vi "RT TDMS buffer and interpolate.vi"(0 "State Info":T4, 7 "TDMS config":T1, 11 "error in":errorcluster, 13 "Operation":T3(ring)) -> (4 "State Info out":T2, 15 "error out":errorcluster)   [LabVIEW 2010, in "TDMS Custom Device.lvlib"]
uses:
  TDMS Custom Device.lvlib
  <vilib>/Analysis/NI_AALPro.lvlib
  <vilib>/gmath/NI_Gmath.lvlib
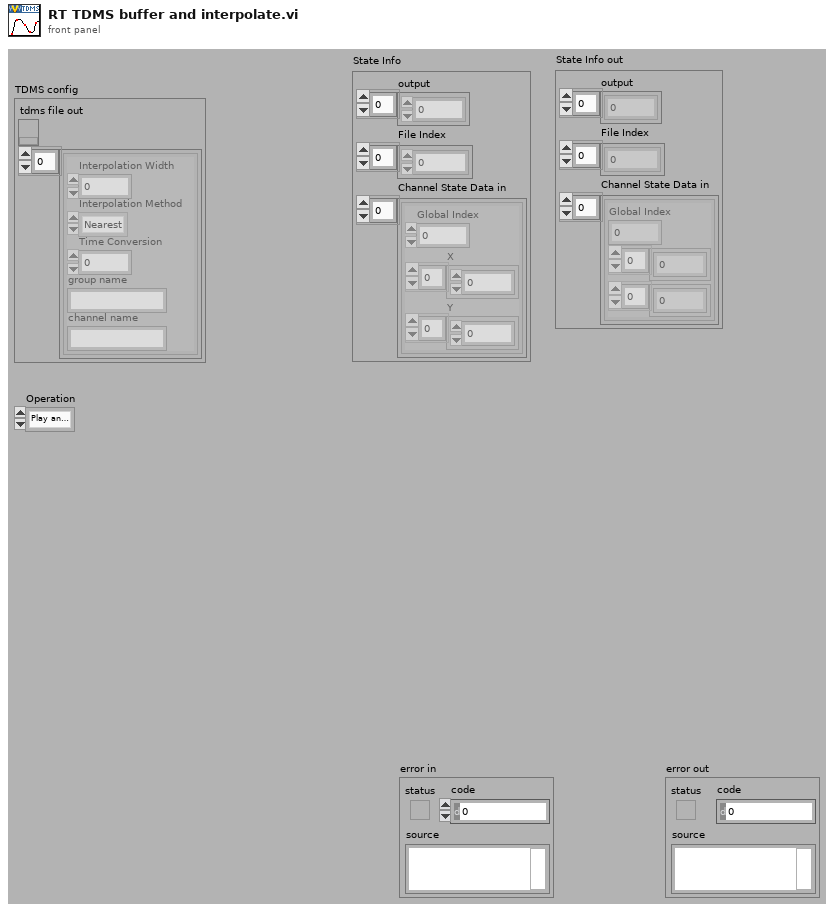
[diagram p1: front panel]
types:
  T1 = cluster{"tdms file out":refnum<k34>, cluster{"Interpolation Width":i32, "Interpolation Method":enum16{"Nearest", "Linear", "Spline", "Cubic Hermite", "Lagrange", "Polynomial"}, "Time Conversion":dbl, "group name":string, "channel name":string}[]}
  T2 = cluster{"output":dbl[], "File Index":i64[], "Channel State Data in":cluster{"Global Index":i64, dbl[], dbl[]}[]}
  T3 = enum16{"Play and Repeat Last", "Stop (and Reset)", "Loop", "Pause"}
  T4 = cluster{"output":dbl[], "File Index":i64[], "Channel State Data in":cluster{"Global Index":i64, "X":dbl[], "Y":dbl[]}[]}
  T5 = cluster{"Global Index":i64, "X":dbl[], "Y":dbl[]}[]
  T6 = cluster{"Interpolation Width":i32, "Interpolation Method":enum16{"Nearest", "Linear", "Spline", "Cubic Hermite", "Lagrange", "Polynomial"}, "Time Conversion":dbl, "group name":string, "channel name":string}[]
  T7 = enum16{"Nearest", "Linear", "Spline", "Cubic Hermite", "Lagrange", "Polynomial"}
  T8 = cluster{"Global Index":i64, "X":dbl[], "Y":dbl[]}
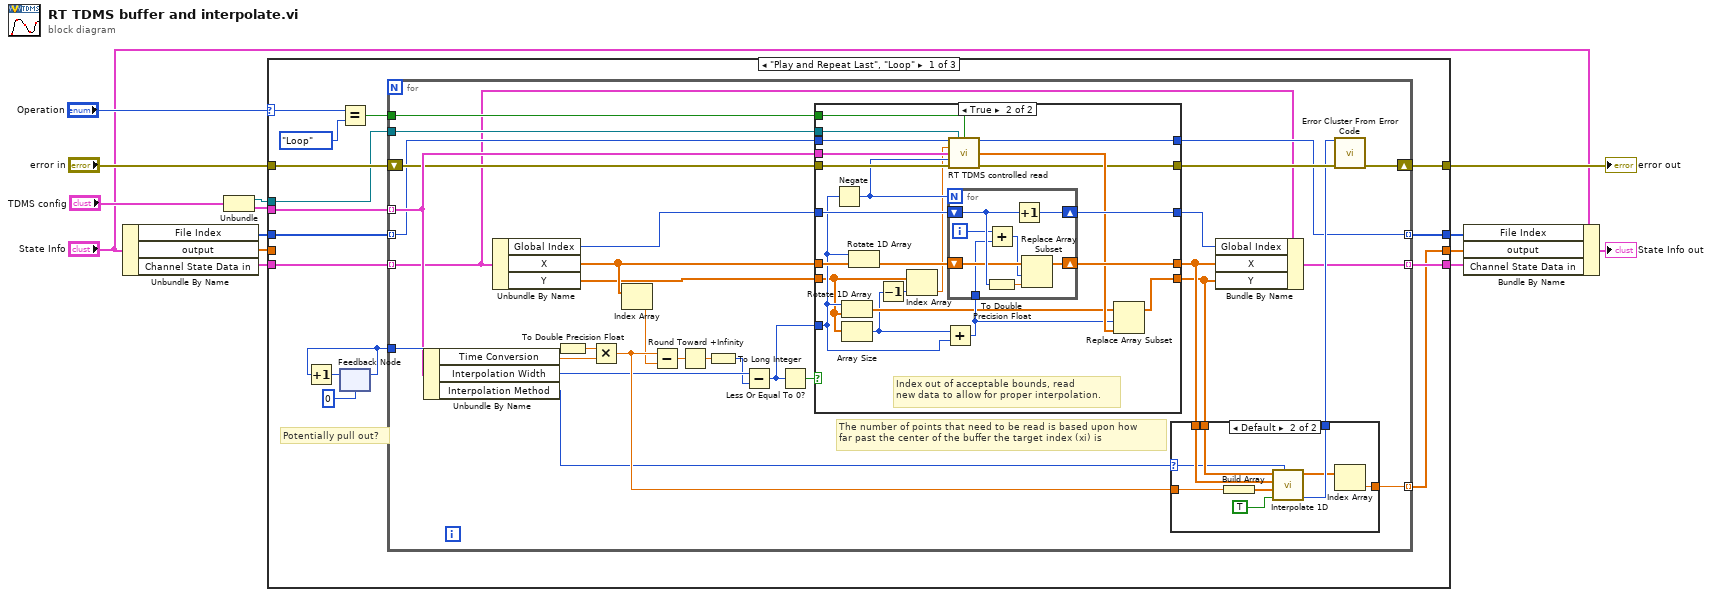
[diagram p0: block diagram]
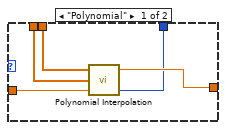
[diagram p2: hidden frame]
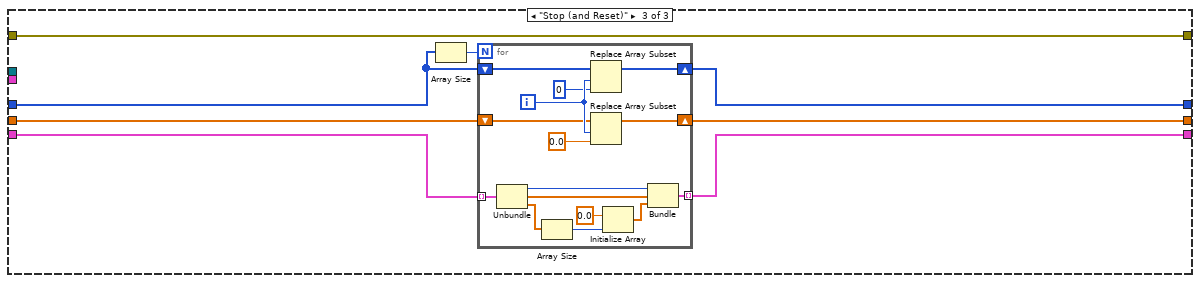
[diagram p5: hidden frame]
diagram:
  n1 = Unbundle By Name("State Info") -> ("File Index"=w8:i64[], "output"=w9:dbl[], "Channel State Data in"=w10:T5)
  n2 = Unbundle("TDMS config") -> ("tdms file out"=w1:refnum<k34>, w2:T6)
  n3 = case shown="\"Play and Repeat Last\", \"Loop\"" "Operation" {
    selector: "Operation" -> [w20 _ _]
    tunnel: "error in" -> [w29 w109 w120]
    tunnel: [w28 w109 w120] -> w13
    tunnel: w9 -> [_ w111 w119]
    tunnel: w2 -> [w27 _ _]
    tunnel: w1 -> [w26 _ _]
    tunnel: w8 -> [w17 w112 w117]
    tunnel: w10 -> [w25 w110 w114]
    tunnel: [w24 w110 w113] -> w7
    tunnel: [w15 w111 w116] -> w3
    tunnel: [w16 w112 w115] -> w4
    frame "Play and Repeat Last", "Loop" {
      # "Potentially pull out?"
      n4 = Equal?(x=w20, y=T3."Loop" ("element")) -> (x = y?=w18:bool)
      n5 = feedback #1(i64 0 ("System Time Index 2")) -> (w21:i64)
      n6 = Increment(x=w21) -> (x+1=w22:i64)
      n7 = feedback-in #1(w22) -> ()
      n8 = for {
        tunnel: w25 -> [w36] mode=indexing
        tunnel: w21 -> [w59]
        tunnel: w27 -> [w56] mode=indexing
        tunnel: [w57] -> w15 mode=indexing
        shift-right: [w53] -> w28
        shift-left: w29 -> [w55]
        tunnel: w26 -> [w51]
        tunnel: w17 -> [w50] mode=indexing
        tunnel: [w35] -> w24 mode=indexing
        tunnel: [w48] -> w16 mode=indexing
        tunnel: w18 -> [w49]
        # "The number of points that need to be read is based upon how\nfar past the center of the buffer the target index (xi) is"
        n9 = Unbundle By Name(w56) -> ("Time Conversion"=w45:dbl, "Interpolation Width"=w31:i32, "Interpolation Method"=w42:T7)
        n10 = Unbundle By Name(w36) -> ("Global Index"=w39:i64, "X"=w38:dbl[], "Y"=w37:dbl[])
        n11 = To Double Precision Float(number=w59) -> (double precision float=w58:dbl)
        n12 = Multiply(x=w58, y=w45) -> (x*y=w47:dbl)
        n13 = Index Array(array=w38) -> (element=w46:dbl)  [unwired: 1 in]
        n14 = Subtract(x=w47, y=w46) -> (x-y=w44:dbl)
        n15 = Round Toward +Infinity(x=w44) -> (ceil(x): smallest int >= x=w43:dbl)
        n16 = To Long Integer(number=w43) -> (32bit integer=w30:i32)
        n17 = Subtract(x=w31, y=w30) -> (x-y=w40:i32)
        n18 = Less Or Equal To 0?(x=w40) -> (x <= 0?=w41:bool)
        n19 = case shown="True" w41 {
          tunnel: w37 -> [w78 w82]
          tunnel: [w74 w100] -> w33
          tunnel: [w78 w99] -> w32
          tunnel: [w75 w98] -> w34
          tunnel: w39 -> [w75 w97]
          tunnel: w56 -> [_ w95]
          tunnel: w40 -> [_ w85]
          tunnel: w50 -> [w76 w87]
          tunnel: [w77 w94] -> w54
          tunnel: w55 -> [w77 w93]
          tunnel: [w76 w92] -> w48
          tunnel: w38 -> [w74 w91]
          tunnel: w51 -> [_ w79]
          tunnel: w49 -> [_ w90]
          frame False {
            # "Index within acceptable bounds, read nothing."
          }
          frame True {
            # "Index out of acceptable bounds, read\nnew data to allow for proper interpolation."
            n20 = Negate(x=w85) -> (-x=w88:i32)
            n21 = Rotate 1D Array(1:w82, 2:w85) -> (0:w83:dbl[])
            n22 = Array Size(array=w82) -> (size(s)=w80:i32)
            n23 = Rotate 1D Array(1:w91, 2:w85) -> (0:w89:dbl[])
            n24 = Decrement(x=w80) -> (x-1=w81:i32)
            n25 = Index Array(array=w82, index=w81) -> (element=w84:dbl)
            n26 = Add(x=w80, y=w85) -> (x+y=w86:i32)
            n27 = for {
              N: w88 -> [_]
              shift-right: [w104] -> w100
              shift-left: w89 -> [w106]
              shift-right: [w107] -> w98
              shift-left: w97 -> [w108]
              tunnel: w86 -> [w101]
              i -> [w102]
              n28 = Add(x=w102, y=w101) -> (x+y=w103:i32)
              n29 = To Double Precision Float(number=w108) -> (double precision float=w105:dbl)
              n30 = Increment(x=w108) -> (x+1=w107:i64)
              n31 = Replace Array Subset(array=w106, new element=w105, index=w103) -> (w104:dbl[])
            }
            n32 = call "RT TDMS controlled read.vi"("start index"=w87, "tdms file"=w79, "loop at EOF?"=w90, "Last Output"=w84, "TDMS config"=w95, "Sample Size"=w88, "error in"=w93) -> ("next index"=w92:i64, "new elements"=w96:dbl[], "error out"=w94:errorcluster)  [unwired: 6 out]
            n33 = Replace Array Subset(array=w83, new element=w96, index=w86) -> (w99:dbl[])
          }
        }
        n34 = case shown="Default" w42 {
          selector: w42 -> [_ w65]
          tunnel: w33 -> [w63 w72]
          tunnel: w32 -> [w64 w71]
          tunnel: w47 -> [w62 w70]
          tunnel: [w61 w69] -> w57
          tunnel: [w60 w67] -> w52
          frame "Polynomial" {
            n35 = call <vilib>:"Polynomial Interpolation.vi"("x value"=w62, "X"=w63, "Y"=w64) -> ("error"=w60:i32, "interpolation value"=w61:dbl)  [unwired: 1 out]
          }
          frame Default {
            n36 = Build Array(w70) -> (w73:dbl[])
            n37 = call <vilib>:"Interpolate 1D.vi"("method"=w65, "X is monotonic"=TRUE, "xi"=w73, "X"=w72, "Y"=w71) -> ("error"=w67:i32, "yi"=w66:dbl[])  [unwired: 1 in, 4 out]
            n38 = Index Array(array=w66) -> (element=w69:dbl)  [unwired: 1 in]
          }
        }
        n39 = Bundle By Name(cluster=w36, "Global Index"=w34, "X"=w33, "Y"=w32) -> (w35:T8)
        n40 = call <vilib>:"Error Cluster From Error Code.vi"("error in (no error)"=w54, "error code (0)"=w52) -> ("error out"=w53:errorcluster)  [unwired: 1 in, 6 out]
      }
    }
    frame "Pause" {
    }
    frame "Stop (and Reset)" {
      n41 = Array Size(array=w117) -> (size(s)=w118:i32)
      n42 = for {
        N: w118 -> [_]
        shift-right: [w131] -> w115
        shift-left: w117 -> [w135]
        shift-right: [w132] -> w116
        shift-left: w119 -> [w133]
        tunnel: w114 -> [w130] mode=indexing
        tunnel: [w129] -> w113 mode=indexing
        i -> [w134]
        n43 = Unbundle(w130) -> ("Global Index"=w124:i64, "X"=w123:dbl[], "Y"=w125:dbl[])
        n44 = Array Size(array=w125) -> (size(s)=w127:i32)
        n45 = Replace Array Subset(array=w135, new element=i64 0 ("new element/subarray"), index=w134) -> (w131:i64[])
        n46 = Replace Array Subset(array=w133, new element=0.0 ("new element/subarray"), index=w134) -> (w132:dbl[])
        n47 = Initialize Array(0.0 ("element"), w127) -> (w126:dbl[])
        n48 = Bundle("Global Index"=w124, "X"=w123, w126) -> (w129:cluster{"Global Index":i64, "X":dbl[], dbl[]})  [unwired: 1 out]
      }
    }
  }
  "error out" <- w13
  n49 = Bundle By Name(cluster="State Info", "File Index"=w4, "output"=w3, "Channel State Data in"=w7) -> (→"State Info out":T4)
